vi "PointAndMotion.vi"(8 "Motion Points":u32, 9 "Motion Increment":u32, 10 "Num Points":u32, 11 "Sample Num":u32) -> (0 "Motion Frame":u32, 1 "Rep Num":u32, 2 "Point Num":u32, 3 "Point Location":u32)   [LabVIEW 2012]
doc: "Computes the memory location for a given sample number to multiplex between motion tracking and point scanning."
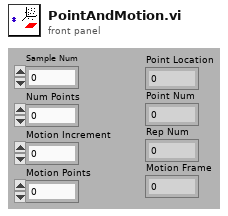
[diagram p1: front panel]
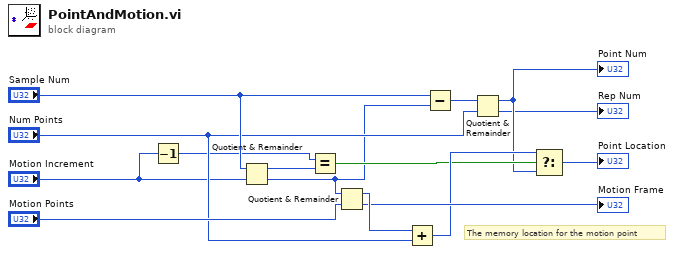
[diagram p0: block diagram]
diagram:
  # "The memory location for the motion point"
  n1 = Decrement(x="Motion Increment") -> (x-1=w2:u32)
  n2 = Quotient & Remainder(x="Sample Num", y="Motion Increment") -> (x-y*floor(x/y)=w15:u32, floor(x/y)=w1:u32)
  n3 = Equal?(x=w2, y=w15) -> (x = y?=w7:bool)
  n4 = Quotient & Remainder(x=w1, y="Motion Points") -> (x-y*floor(x/y)=w13:u32, floor(x/y)=→"Motion Frame":u32)
  n5 = Add(x=w13, y="Num Points") -> (x+y=w11:u32)
  n6 = Subtract(x="Sample Num", y=w1) -> (x-y=w9:u32)
  n7 = Quotient & Remainder(x=w9, y="Num Points") -> (x-y*floor(x/y)=w6:u32, floor(x/y)=→"Rep Num":u32)
  "Point Num" <- w6
  n8 = Select(t=w11, s=w7, f=w6) -> (s? t:f=→"Point Location":u32)
